vi "GetXML.vi"(3 "Baxter":T2, 4 "topic port":u16, 5 "Connections":T1(array[cluster]), 6 "connection ID in":refnum<k5>) -> (0 "error IO":errorcluster, 1 "Subscribers":T1(array[cluster]), 2 "connection ID out":refnum<k5>)   [LabVIEW 2010]
uses:
  <userlib>/ROSforLV_0.1/ROS/Code/SubVIs/_ROSControl.ctl
  <userlib>/ROSforLV_0.1/ROS/Code/SubVIs/_ROSDirection.ctl
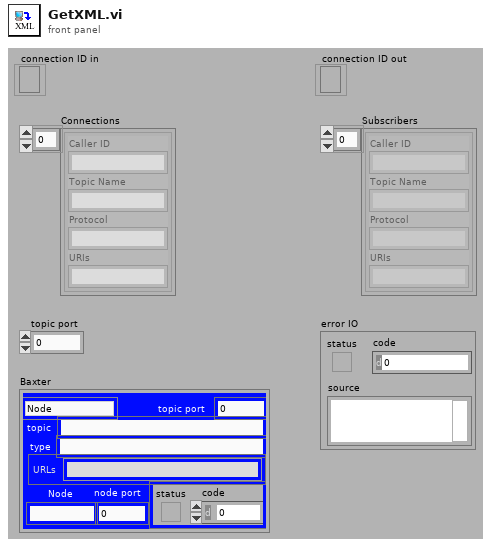
[diagram p1: front panel]
types:
  T1 = cluster{"Caller ID":string, "Topic Name":string, "Protocol":string, "URIs":string}[]
  T2 = typedef "_ROSControl.ctl" = cluster{"topic port":u16, "Node":string, "topic":string, "type":string, "node port":u32, "error ":errorcluster, "Direction":T3, "APIs":string[]}
  T3 = typedef "_ROSDirection.ctl" = enum16{"Node", "Publisher", "Subscriber", "Service Client"}
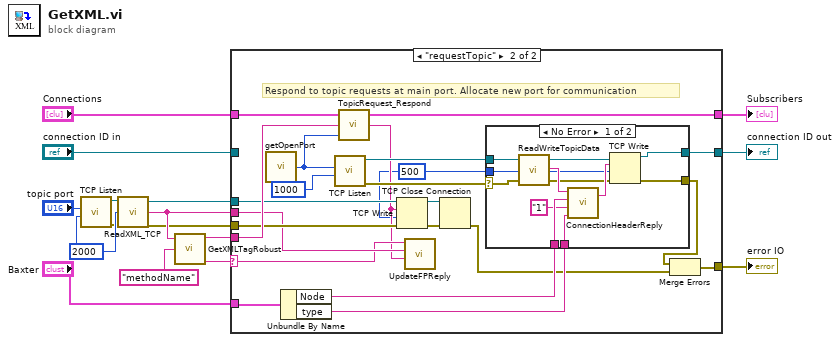
[diagram p0: block diagram]
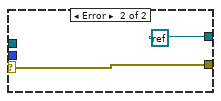
[diagram p3: hidden frame]
diagram:
  w16 = 2000 ("timeout ms (wait forever: -1)")
  n1 = call <vilib>:"TCP Listen.vi"("timeout ms (wait forever: -1)"=w16, "port"="topic port") -> ("error out"=w15:errorcluster, "connection ID"=w14:refnum<k5>)  [unwired: 6 in, 2 out]
  n2 = call <userlib>:"ReadXML_TCP.vi"("error in"=w15, "timeout ms (3000)"=w16, "connection ID in"=w14) -> ("error out"=w6:errorcluster, "data out"=w10:string, "connection ID out"=w5:refnum<k5>)
  n3 = call <userlib>:"GetXMLTagRobust.vi"("Tag"="methodName", "String"=w10) -> ("value"=w2:string, "String w/o Tag"=w3:string)  [unwired: 1 in, 2 out]
  n4 = case shown="\"requestTopic\"" w2 {
    selector: w2 -> [_ w28]
    tunnel: w3 -> [_ w41]
    tunnel: "Connections" -> [w19 w25]
    tunnel: w5 -> [_ w38]
    tunnel: w6 -> [w17 w37]
    tunnel: [w19 w39] -> w7
    tunnel: [w18 w26] -> w8
    tunnel: "connection ID in" -> [w18 _]
    tunnel: "Baxter" -> [_ w32]
    tunnel: w10 -> [_ w29]
    tunnel: [w17 w21] -> w11
    frame Default {
    }
    frame "requestTopic" {
      w24 = 500 ("timeout ms (25000)")
      # "Respond to topic requests at main port. Allocate new port for communication"
      n5 = call <userlib>:"getOpenPort.vi"() -> ("port"=w40:u16)
      n6 = Unbundle By Name(w32) -> ("Node"=w31:string, "type"=w30:string)
      n7 = call <vilib>:"TCP Listen.vi"("timeout ms (wait forever: -1)"=1000, "port"=w40) -> ("error out"=w34:errorcluster, "connection ID"=w33:refnum<k5>)  [unwired: 6 in, 2 out]
      n8 = call <userlib>:"TopicRequest_Respond.vi"("port"=w40, "XML"=w41, "Subscribers"=w25) -> ("Topic Request Reply"=w27:string, "Subscribers"=w39:T1)  [unwired: 1 in]
      n9 = TCP Write(connection ID=w38, data in=w27, error in (no error)=w37, 9:w24) -> (connection ID out=w35:refnum<k5>, error out=w36:errorcluster)  [unwired: 1 out]
      n10 = call <userlib>:"UpdateFPReply.vi"("Reply"=w27, "Sent"=w29, "method"=w28) -> ()  [unwired: 3 in]
      n11 = TCP Close Connection(connection ID=w35, error in (no error)=w36) -> (error out=w23:errorcluster)  [unwired: 1 in, 1 out]
      n12 = case shown="No Error" w34 {
        selector: w34 -> [w52 w54]
        tunnel: w33 -> [w53 _]
        tunnel: w31 -> [w50 _]
        tunnel: w30 -> [w48 _]
        tunnel: [w45 refnum<k0> refnum] -> w26
        tunnel: [w43 w54] -> w22
        tunnel: w24 -> [w42 _]
        frame No Error {
          n13 = call <userlib>:"ReadWriteTopicData.vi"("error in (no error)"=w52, "timeout ms (1000)"=w42, "connection ID in"=w53) -> ("error out"=w44:errorcluster, "data out"=w51:string, "connection ID out"=w46:refnum<k5>)
          n14 = call <userlib>:"ConnectionHeaderReply.vi"("type"=w48, "Latching"="1", "Caller ID"=w50, "TCPROS Connection Header"=w51) -> ("Connection Response"=w47:string)  [unwired: 1 in]
          n15 = TCP Write(connection ID=w46, data in=w47, error in (no error)=w44, 9:w42) -> (connection ID out=w45:refnum<k5>, error out=w43:errorcluster)  [unwired: 1 out]
        }
        frame Error {
        }
      }
      n16 = Merge Errors(w22, w23) -> (w21:errorcluster)
    }
  }
  "error IO" <- w11
  "connection ID out" <- w8
  "Subscribers" <- w7
